vi "Merge.vi"(4 "Second Error In":refnum<class "MultiErrors.lvclass">, 5 "First Error In":refnum<class "MultiErrors.lvclass">) -> (7 "MultiErrors out":refnum<class "MultiErrors.lvclass">)   [LabVIEW 2020, in "Volatus.lvlib" / "MultiErrors.lvclass"]
uses:
  MultiErrors.lvclass
  MultiErrors.lvclass/MultiErrors.ctl
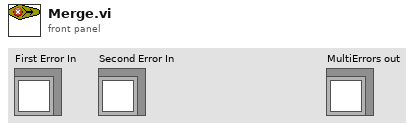
[diagram p1: front panel]
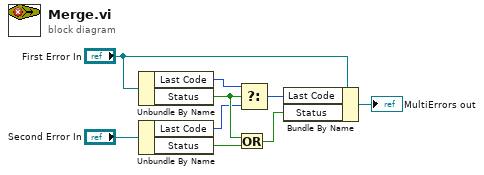
[diagram p0: block diagram]
diagram:
  n1 = Unbundle By Name("First Error In") -> ("Last Code"=w6:i32, "Status"=w7:bool)
  n2 = Unbundle By Name("Second Error In") -> ("Last Code"=w5:i32, "Status"=w8:bool)
  n3 = Or(x=w7, y=w8) -> (x .or. y?=w2:bool)
  n4 = Select(t=w6, s=w7, f=w5) -> (s? t:f=w3:i32)
  n5 = Bundle By Name(cluster="First Error In", "Last Code"=w3, "Status"=w2) -> (→"MultiErrors out":refnum<class "MultiErrors.lvclass">)
